vi "PH_Interaction.get Vision IDs on same Node.vi"(3 "Cam Instances":string[](array[string]), 5 "i ref in":refnum<vi>) -> (0 "Vision System IDs":string[](array[string]), 1 "Vision Sytem IDs found":bool, 2 "Cams instanciated on own system":bool)   [LabVIEW 2014, in "PH_Common.lvlib"]
doc: "This VI checks whether the list of connected cams is running at the same node, and if, whether they are running at different system IDs."
uses:
  PH_Common.lvlib
  CSCore/CSSystem/CSSystemLib/CSSystemLib.lvlib
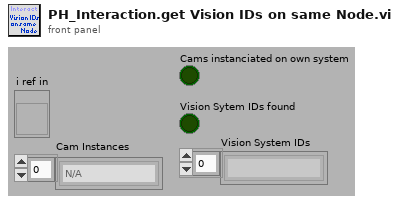
[diagram p1: front panel]
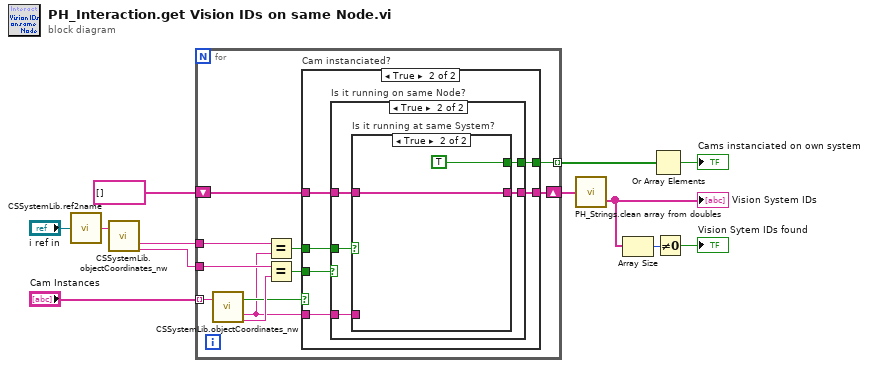
[diagram p0: block diagram]
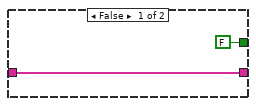
[diagram p2: hidden frame]
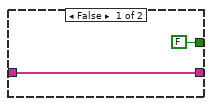
[diagram p3: hidden frame]
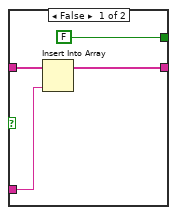
[diagram p4: hidden frame]
diagram:
  n1 = call "CSSystemLib.ref2name.vi"("obj refnum"="i ref in") -> ("name"=w11:string)
  n2 = call "CSSystemLib.objectCoordinates_nw.vi"("name"=w11) -> ("systemID"=w10:string, "node"=w9:string)  [unwired: 15 in, 2 out]
  n3 = for {
    tunnel: "Cam Instances" -> [w20] mode=indexing
    tunnel: w10 -> [w19]
    tunnel: w9 -> [w18]
    shift-right: [w14] -> w7
    shift-left: string[] [] -> [w15]
    tunnel: [w13] -> w2 mode=indexing
    n4 = call "CSSystemLib.objectCoordinates_nw.vi"("name"=w20) -> ("obj exists"=w21:bool, "systemID"=w16:string, "node"=w23:string)  [unwired: 15 in, 1 out]
    n5 = Equal?(x=w19, y=w16) -> (x = y?=w17:bool)
    n6 = Equal?(x=w18, y=w23) -> (x = y?=w22:bool)
    n7 = case "Cam instanciated?" shown="True" w21 {
      tunnel: w22 -> [_ w31]
      tunnel: w17 -> [_ w30]
      tunnel: w16 -> [_ w29]
      tunnel: w15 -> [w25 w28]
      tunnel: [w25 w27] -> w14
      tunnel: [FALSE w26] -> w13
      frame False {
      }
      frame True {
        n8 = case "Is it running on same Node?" shown="True" w31 {
          tunnel: w30 -> [_ w38]
          tunnel: w29 -> [_ w37]
          tunnel: w28 -> [w33 w36]
          tunnel: [w33 w35] -> w27
          tunnel: [FALSE w34] -> w26
          frame False {
          }
          frame True {
            n9 = case "Is it running at same System?" shown="True" w38 {
              tunnel: w37 -> [w42 _]
              tunnel: w36 -> [w41 w44]
              tunnel: [w40 w44] -> w35
              tunnel: [FALSE TRUE] -> w34
              frame False {
                n10 = Insert Into Array(array=w41, new element=w42) -> (w40:string[])  [unwired: 1 in]
              }
              frame True {
              }
            }
          }
        }
      }
    }
  }
  n11 = call "PH_Strings.clean array from doubles.vi"("Array Input"=w7) -> ("Cleaned Array Output"=w6:string[])  [unwired: 1 out]
  "Vision System IDs" <- w6
  n12 = Array Size(array=w6) -> (size(s)=w5:i32)
  n13 = Or Array Elements(Boolean array=w2) -> (logical OR=→"Cams instanciated on own system":bool)
  n14 = Not Equal To 0?(x=w5) -> (x != 0?=→"Vision Sytem IDs found":bool)
